vi "SetStagePosition.vi"(0 "Microscope in":refnum<class "Microscope.lvclass">, 5 "Label":string, 7 "AbsPosition?":bool=TRUE, 9 "Value":dbl format="%#_13g", 11 "error in (no error)":errorcluster) -> (4 "Microscope out":refnum<class "Microscope.lvclass">, 15 "error out":errorcluster)   [LabVIEW 2020, in "Microscope.lvlib" / "Microscope.lvclass"]
uses:
  Microscope.lvclass
  Microscope.lvclass/Microscope.ctl
  Component/Stage/Stage Messages/SetRelativePositionUm Msg/SetRelativePositionUm Msg.lvclass/SetRelativePositionUm Msg.ctl
  <vilib>/ActorFramework/Message Enqueuer/Message Enqueuer.lvclass/Message Enqueuer.ctl
  Component/Stage/Stage Messages/SetPositionUm Msg/SetPositionUm Msg.lvclass/SetPositionUm Msg.ctl
  <vilib>/ActorFramework/Message Enqueuer/Enqueue.vi
  Component/Stage/Stage Messages/SetRelativePositionUm Msg/SetRelativePositionUm Msg.lvclass
  C:/Program Files/National Instruments/LabVIEW 2020/vi.lib/ActorFramework/Message/Message.lvclass
  Component/Stage/Stage Messages/SetPositionUm Msg/SetPositionUm Msg.lvclass
  <vilib>/ActorFramework/Message Priority Queue/Priority Enqueue.vi
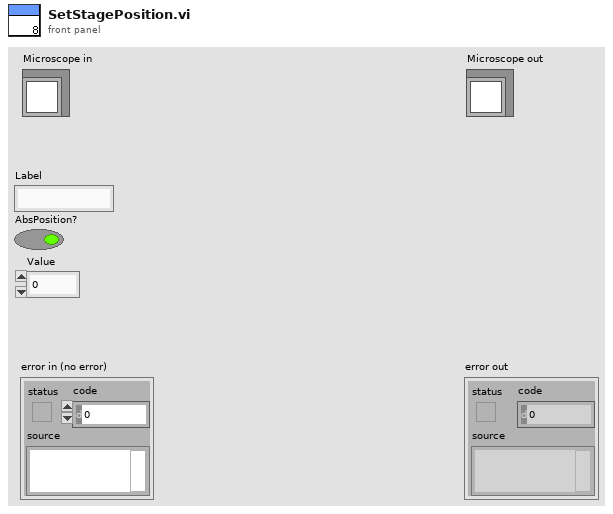
[diagram p1: front panel]
types:
  T1 = map{string, refnum<class "Message Enqueuer.lvclass">}
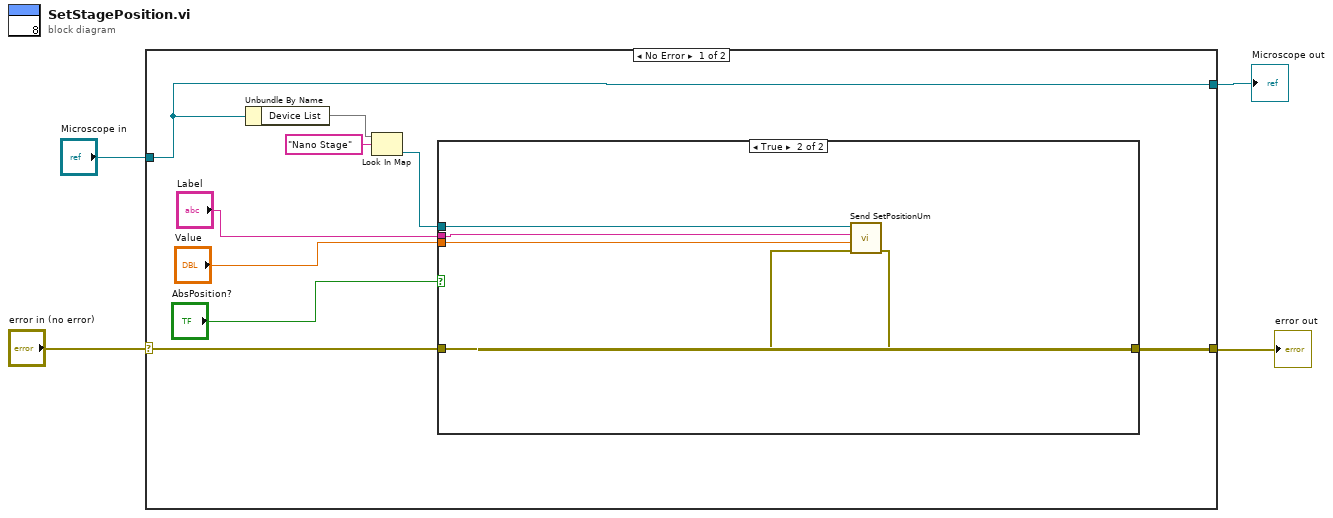
[diagram p0: block diagram]
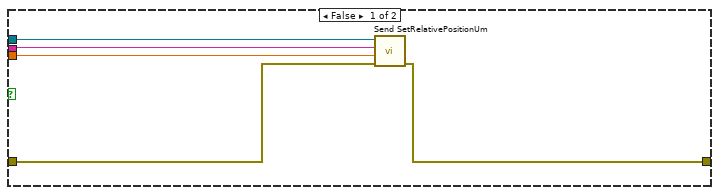
[diagram p2: hidden frame]
diagram:
  n1 = case shown="No Error" "error in (no error)" {
    selector: "error in (no error)" -> [w6 w24]
    tunnel: [w5 w24] -> w3
    tunnel: "Microscope in" -> [w12 w25]
    tunnel: [w12 w25] -> w1
    frame No Error {
      n2 = Unbundle By Name(w12) -> ("Device List"=w11:T1)
      n3 = Look In Map(map=w11, key="Nano Stage") -> (value=w9:refnum<class "Message Enqueuer.lvclass">)  [unwired: 1 in, 1 out]
      n4 = case shown="True" "AbsPosition?" {
        tunnel: w9 -> [w18 w23]
        tunnel: "Label" -> [w17 w22]
        tunnel: "Value" -> [w16 w21]
        tunnel: w6 -> [w15 w20]
        tunnel: [w14 w19] -> w5
        frame False {
          n5 = call "Send SetRelativePositionUm.vi"("error in (no error)"=w15, "RelativeMoveum"=w16, "Stage Label"=w17, "Message Enqueuer"=w18) -> ("error out"=w14:errorcluster)  [unwired: 6 in, 1 out]
        }
        frame True {
          n6 = call "Send SetPositionUm.vi"("error in (no error)"=w20, "Positionum"=w21, "Stage Label"=w22, "Message Enqueuer"=w23) -> ("error out"=w19:errorcluster)  [unwired: 6 in, 1 out]
        }
      }
    }
    frame Error {
    }
  }
  "error out" <- w3
  "Microscope out" <- w1
